vi "LVCAM Write LVCAM.vi"(10 "LVCAM":refnum<class "LVCAM.lvclass">, 11 "LVCAM Write LVCAM in":refnum<class "LVCAM Write LVCAM.lvclass">) -> (3 "LVCAM Write LVCAM out":refnum<class "LVCAM Write LVCAM.lvclass">)   [LabVIEW 2021, in "LVCAM.lvlib" / "LVCAM Write LVCAM.lvclass"]
uses:
  LVCAM Write LVCAM.lvclass
  LVCAM/LVCAM.lvclass
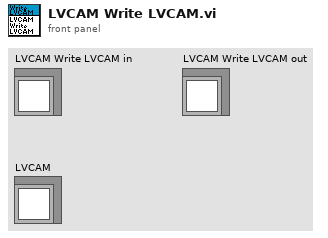
[diagram p1: front panel]
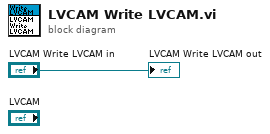
[diagram p0: block diagram]
diagram:
  "LVCAM Write LVCAM out" <- "LVCAM Write LVCAM in"
